vi "SSC DAQmx Calculate Per-Site Per-Pin to Per-Instrument LUT.vi"(0 "DAQmx SSC in":T1[](array[typedef]), 7 "Sites":i32[](array[numeric]), 9 "Pins":tag[](array[tag]), 11 "AO Channels":refnum<k21>[][](array[refnum])) -> (4 "Per-Site Per-Pin to Per-Task LUT":T2[][](array[typedef]), 6 "Task Count":i32, 8 "Max Channels in a Task":i32)   [LabVIEW 2020]
uses:
  Digital/SubVIs/Digital 2D Location.ctl
  Pin Map/SSC DAQmx.ctl
  Shared SubVIs/Trim Whitespace [Inlined].vi
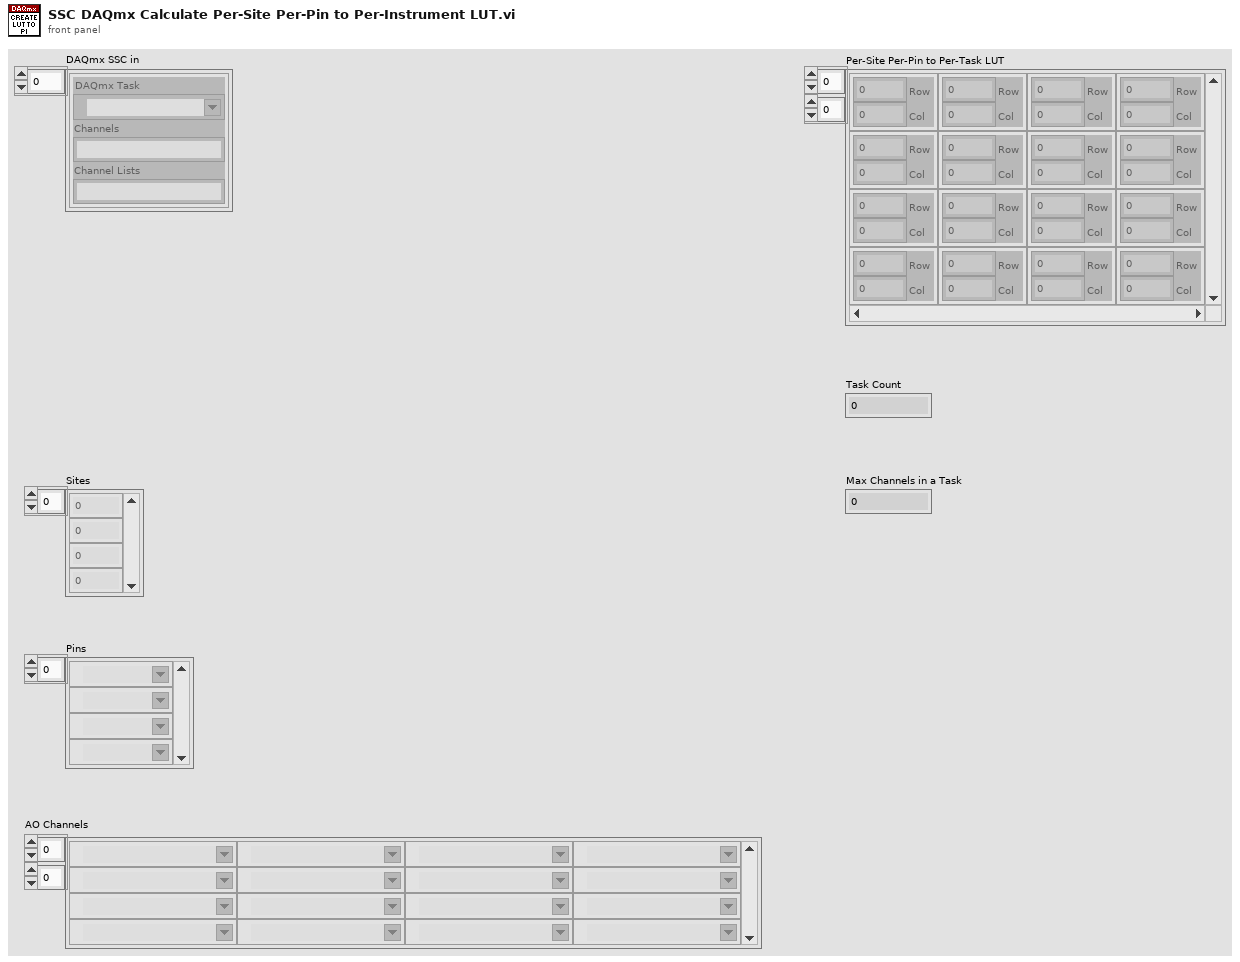
[diagram p1: front panel]
types:
  T1 = typedef "SSC DAQmx.ctl" = cluster{"DAQmx Task ":refnum<k21>, "Channels":string, "Channel Lists":string}
  T2 = typedef "Digital 2D Location.ctl" = cluster{"Row":i32, "Col":i32}
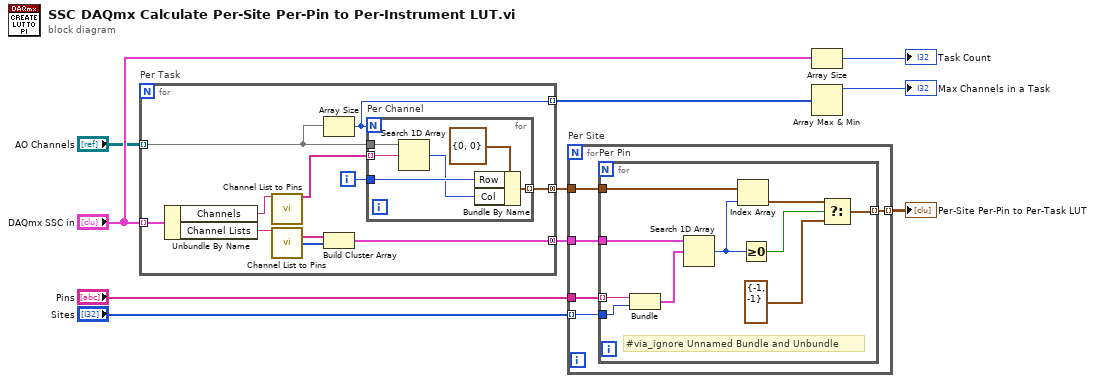
[diagram p0: block diagram]
diagram:
  n1 = for "Per Task" {
    tunnel: "DAQmx SSC in" -> [w21] mode=indexing
    tunnel: [w18] -> w7 mode=concatenating
    tunnel: [w15] -> w6 mode=concatenating
    tunnel: [w14] -> w3 mode=indexing
    tunnel: "AO Channels" -> [w11] mode=indexing
    i -> [w16]
    n2 = Unbundle By Name(w21) -> ("Channels"=w13:string, "Channel Lists"=w20:string)
    n3 = call "Channel List to Pins.vi"("Channel List"=w13) -> ("Sites and Pins"=w12:string[])  [unwired: 12 in, 2 out]
    n4 = call "Channel List to Pins.vi"("Channel List"=w20) -> ("Pins"=w17:tag[], "Sites"=w19:i32[])  [unwired: 12 in, 1 out]
    n5 = Array Size(array=w11) -> (size(s)=w14:i32)
    n6 = Build Cluster Array(w17, w19) -> (w18:cluster{"Pin":tag, "trimmed string":i32}[])
    n7 = for "Per Channel" {
      N: w14 -> [_]
      tunnel: w16 -> [w25]
      tunnel: [w26] -> w15 mode=indexing
      tunnel: w11 -> [w24]
      tunnel: w12 -> [w23] mode=indexing
      n8 = Search 1D Array(1D array=w24, element=w23) -> (index of element=w22:i32)  [unwired: 1 in]
      n9 = Bundle By Name(cluster=T2 {"Row"=0, "Col"=0}, "Row"=w25, "Col"=w22) -> (w26:T2)
    }
  }
  n10 = for "Per Site" {
    tunnel: "Sites" -> [w30] mode=indexing
    tunnel: "Pins" -> [w31]
    tunnel: [w32] -> w8 mode=indexing
    tunnel: w7 -> [w29]
    tunnel: w6 -> [w28]
    n11 = for "Per Pin" {
      tunnel: [w36] -> w32 mode=indexing
      tunnel: w31 -> [w41] mode=indexing
      tunnel: w30 -> [w40]
      tunnel: w29 -> [w42]
      tunnel: w28 -> [w38]
      # "#via_ignore Unnamed Bundle and Unbundle"
      n12 = Bundle("Pin"=w41, "Site Number"=w40) -> (w39:cluster{"Pin":tag, "Site Number":i32})  [unwired: 1 in]
      n13 = Search 1D Array(1D array=w42, element=w39) -> (index of element=w35:i32)  [unwired: 1 in]
      n14 = Index Array(array=w38, index=w35) -> (element=w37:T2)
      n15 = Greater Or Equal To 0?(x=w35) -> (x >= 0?=w34:bool)
      n16 = Select(t=w37, s=w34, f=T2 {"Row"=-1, "Col"=-1}) -> (s? t:f=w36:T2)
    }
  }
  "Per-Site Per-Pin to Per-Task LUT" <- w8
  n17 = Array Size(array="DAQmx SSC in") -> (size(s)=→"Task Count":i32)
  n18 = Array Max & Min(array=w3) -> (max value=→"Max Channels in a Task":i32)  [unwired: 3 out]
